vi "SignalGenerator.vi"(10 "Amplitude":dbl=1.0, 11 "Frequency":dbl=10.1) -> (1 "Sine":dynamicdata(graph))   [LabVIEW 2015]
panel:
  out "error out":errorcluster
  out "error in":errorcluster caption="error in (no error)"
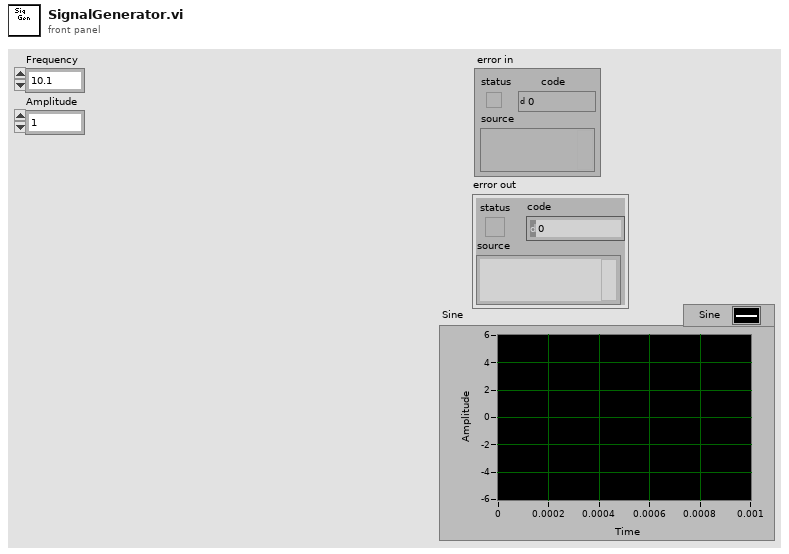
[diagram p1: front panel]
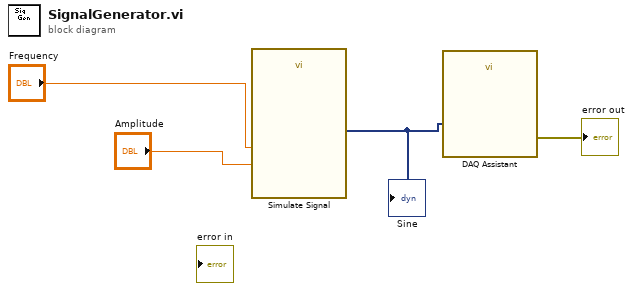
[diagram p0: block diagram]
diagram:
  n1 = call "Simulate Signal"("Frequency"="Frequency", "Amplitude"="Amplitude") -> ("Sine"=w1:dynamicdata)  [unwired: 12 in, 1 out]
  "Sine" <- w1
  n2 = call "DAQ Assistant"("data"=w1) -> ("error out"=→"error out":errorcluster)  [unwired: 17 in, 1 out]
